vi "CAN.Initialize.vi"(8 "error in (no error)":errorcluster, 11 "Parameters":T5={"Name"="", "CAN"={"Interface"="", "Baud Rate"=0, "Diagnostic Protocol"=enum."GMLAN", "Transport Protocol"=enum."ISO TP - Normal Mode", "Transmit ID"=0, "Receive ID"=2, "Transmit Extension"=1, "Receive Extension"=255, "Receive UUDT ID"=0, "Enable Stream"=TRUE, "VW TP Channel ID"=1, "Fill Frame"=FALSE, "Fill Byte"=0, "Termination"=FALSE, "LIN Cluster"="", "NAD"=8, "IO Mode"=0, "Max DLC"=0, "FD Baud Rate"=2, "Timeout"=1}, "986x"={"Enable"=FALSE, "RIO Device"="", "Bitfile"=path ""}, "Reads"=[], "Frames Lookup"=variant(enum16{"GMLAN", "KWP-2000", "UDS"} enum."GMLAN"), "Writes"=[], "DPIDs"=[], "DPID Lookup"=variant(u32 0), "DTC"={"Descriptor"={"DTC Byte Length"=1, "Status Byte Length"=1, "Add Data Byte Length"=1, "Byte Order"=enum."Motorola"}, "Value.Code"=[], "Value.String"=[], "Value.J2012String"=[], "Status.Code"=[], "Status.String"=[]}, "Created DTCs"=0, "Polls"=[], "Service Channels Status Lookup"=variant, "Trigger Lookup"=variant, "Security"={"Type"=enum."None", "Source DLL Path"=path "", "Target DLL Path"=path "", "Security Level"=0}} {"Writes"."Signals"."Byte Order" items=["Little Endian", "Big Endian"]; "Writes"."Signals"."Data Type" items=["Signed", "Unsigned", "IEEE Float"]; "CAN"."IO Mode" items=["CAN 2.0", "CAN FD", "CAN FD+BRS"]; "CAN"."Fill Byte" format="%.0x"; "CAN"."VW TP Channel ID" format="%.0x"; "CAN"."Receive UUDT ID" format="%.0x"; "CAN"."Receive Extension" format="%.0x"; "CAN"."Transmit Extension" format="%.0x"; "CAN"."Receive ID" format="%.0x"; "CAN"."Transmit ID" format="%.0x"; "Reads"."Signals"."Byte Order" items=["Little Endian", "Big Endian"]; "Reads"."Signals"."Data Type" items=["Signed", "Unsigned", "IEEE Float"]}) -> (0 "error out":errorcluster, 1 "ADCS Connection":T22={"Diag CAN Handle"=0, "Transport Protocol"=enum."ISO TP - Normal Mode", "Receive Address Extension"=0, "Transmit Address Extension"=0, "Receive CAN Id"=0, "Transmit CAN Id"=0, "Log Frames ?"=FALSE, "My TP Address"=0, "Other TP Address"=0, "T1"=0, "T2"=0, "T3"=0, "T4"=0, "Tx SN"=0, "Block Size"=0, "Rx SN"=0, "VW TP Initialized?"=FALSE, "Tx block no"=0, "baud rate"=0, "Interface"="", "Channel Diag CAN Handle"=0, "UDP Connection ID"=refnum, "TCP Connection ID"=refnum, "Target IP Addr"=0, "Source Address"=0, "Target Address"=0, "Send Header NACK?"=FALSE, "DLL Handle"=0, "NAD"=0, "Time Stamp read first"=0.0, "Time Stamp read last"=0.0, "Time Stamp write first"=0.0, "Time Stamp write last"=0.0, "Time Stamp write"=0.0, "Time Stamp read"=0.0, " I/O Mode"=0, "FD Baudrate"=0, "TX_DL"=8, "RX_DL"=8, "DoIP Protocol Version"=1, " Selected I/O Mode"=0, "TesterPresent Counter"=0, "TesterPresent Limit"=0, "TesterPresent Tick[ms]"=10, "TesterPresent RequireResponse?"=FALSE, "TesterPresent Stored Ref?"=FALSE, "TesterPresent Message"=[], "TesterPresent Task Handle"=0, "TesterPresent Semaphore"=refnum, "Response Plausibility Check"=1, "Default Version?"=TRUE, "Diagostic Globals"={"Timeout FC (Bs)"=250, "Timeout CF (Cr)"=250, "Timeout Diag Command"=1000, "Receive Block Size (BS)"=0, "Wait Time CF (STmin)"=5, "Max Waits (N_WFTmax)"=10, "Waits to Send (N_WAIT)"=0, "Time between Waits (TW)"=25, "Fill CAN Frames?"=TRUE, "Fill Byte"=255, "Invalid Response as Error?"=FALSE, "Max RspPending Count"=5, "VWTP Command Timeout"=50, "Transport Protocol"=enum."Diagnostics on IP", "Diag CAN Handle"=0, "DLL Handle"=0, "Timeout RspPending"=1000}, "Session-based Properties?"=FALSE} {"Diagostic Globals"."Fill Byte" format="%x"; "TesterPresent Message" format="%.0x"; "Selected I/O Mode" items=["CAN", "CAN FD", "CAN FD+BRS", "ECU Determined"]; "DoIP Protocol Version" items=["2010"=1, "2012"=2]; "RX_DL" items=["8"=8, "12"=12, "16"=16, "20"=20, "24"=24, "32"=32, "48"=48, "64"=64]; "TX_DL" items=["8"=8, "12"=12, "16"=16, "20"=20, "24"=24, "32"=32, "48"=48, "64"=64]; "I/O Mode" items=["CAN", "CAN FD", "CAN FD+BRS", "Not yet determined"]}, 2 "XNET References":T21, 3 "Parameters":T5={"Name"="", "CAN"={"Interface"="", "Baud Rate"=0, "Diagnostic Protocol"=enum."GMLAN", "Transport Protocol"=enum."ISO TP - Normal Mode", "Transmit ID"=0, "Receive ID"=2, "Transmit Extension"=1, "Receive Extension"=255, "Receive UUDT ID"=0, "Enable Stream"=TRUE, "VW TP Channel ID"=1, "Fill Frame"=FALSE, "Fill Byte"=0, "Termination"=FALSE, "LIN Cluster"="", "NAD"=8, "IO Mode"=0, "Max DLC"=0, "FD Baud Rate"=2, "Timeout"=1}, "986x"={"Enable"=FALSE, "RIO Device"="", "Bitfile"=path ""}, "Reads"=[], "Frames Lookup"=variant(enum16{"GMLAN", "KWP-2000", "UDS"} enum."GMLAN"), "Writes"=[], "DPIDs"=[], "DPID Lookup"=variant(u32 0), "DTC"={"Descriptor"={"DTC Byte Length"=1, "Status Byte Length"=1, "Add Data Byte Length"=1, "Byte Order"=enum."Motorola"}, "Value.Code"=[], "Value.String"=[], "Value.J2012String"=[], "Status.Code"=[], "Status.String"=[]}, "Created DTCs"=0, "Polls"=[], "Service Channels Status Lookup"=variant, "Trigger Lookup"=variant, "Security"={"Type"=enum."None", "Source DLL Path"=path "", "Target DLL Path"=path "", "Security Level"=0}} {"Writes"."Signals"."Byte Order" items=["Little Endian", "Big Endian"]; "Writes"."Signals"."Data Type" items=["Signed", "Unsigned", "IEEE Float"]; "CAN"."IO Mode" items=["CAN 2.0", "CAN FD", "CAN FD+BRS"]; "CAN"."Fill Byte" format="%.0x"; "CAN"."VW TP Channel ID" format="%.0x"; "CAN"."Receive UUDT ID" format="%.0x"; "CAN"."Receive Extension" format="%.0x"; "CAN"."Transmit Extension" format="%.0x"; "CAN"."Receive ID" format="%.0x"; "CAN"."Transmit ID" format="%.0x"; "Reads"."Signals"."Byte Order" items=["Little Endian", "Big Endian"]; "Reads"."Signals"."Data Type" items=["Signed", "Unsigned", "IEEE Float"]}, 5 "Stream Refs":T1 {"Termination" items=["Off", "On"]})   [LabVIEW 2019, in "Diagnostics Addon Engine.lvlib"]
uses:
  Diagnostics Addon Engine.lvlib
  Addon Shared/Types/SysDef.Compile.ctl
  Addon Shared/Types/CAN.ctl
  Addon Shared/Types/CAN.Interface.ctl
  Addon Shared/Types/Protocol.ctl
  Addon Shared/Types/Transport.ctl
  Addon Shared/Types/986x.ctl
  Addon Shared/Types/Frame.Compile.ctl
  Addon Shared/Types/Type.ctl
  Addon Shared/Types/Signal.ctl
  Addon Shared/Types/DPID.ctl
  Addon Shared/Types/DPID.Rate.ctl
  Addon Shared/Types/DTC.Settings.ctl
  Addon Shared/Types/DTC.Descriptor.ctl
  Addon Shared/Types/Poll.Compiled.ctl
  Addon Shared/Types/Security.ctl
  Addon Shared/Types/Security.Type.ctl
  <vilib>/Automotive Diagnostic Command Set/Diagnostic Transport.llb/Diag Reference.ctl
  <vilib>/Automotive Diagnostic Command Set/Diagnostic Transport.llb/Transport Protocol Selector.ctl
  <vilib>/Automotive Diagnostic Command Set/Diagnostic Transport.llb/DoIP Protocol Version.ctl
  <vilib>/Automotive Diagnostic Command Set/Diagnostic Transport.llb/Diag Globals.ctl
  Types/XNET.Refs.ctl
  SubModules/CAN-Streaming-Support/Addon/Addon Engine/Types/Engine Stream Refs.ctl
  SubModules/CAN-Streaming-Support/Addon/Addon Shared/Types/Direction Filter.ctl
  SubModules/CAN-Streaming-Support/Addon/Addon Shared/Types/Type Filter.ctl
  SubModules/CAN-Streaming-Support/Addon/Addon Shared/Types/Filter Parameters.ctl
  <vilib>/xnet/xnet.llb/XNET Create Session (Frame Input Queued).vi
  SubModules/CAN-Streaming-Support/Addon/Addon Engine/CAN Stream Support Engine.lvlib
  Addon Shared/Diagnostics Addon Shared.lvlib
  <vilib>/addons/Automotive Diagnostic Command Set/NI_Automotive Diagnostic Command Set.lvlib
  SubModules/CAN-Streaming-Support/Addon/Addon Shared/CAN Stream Support Shared.lvlib
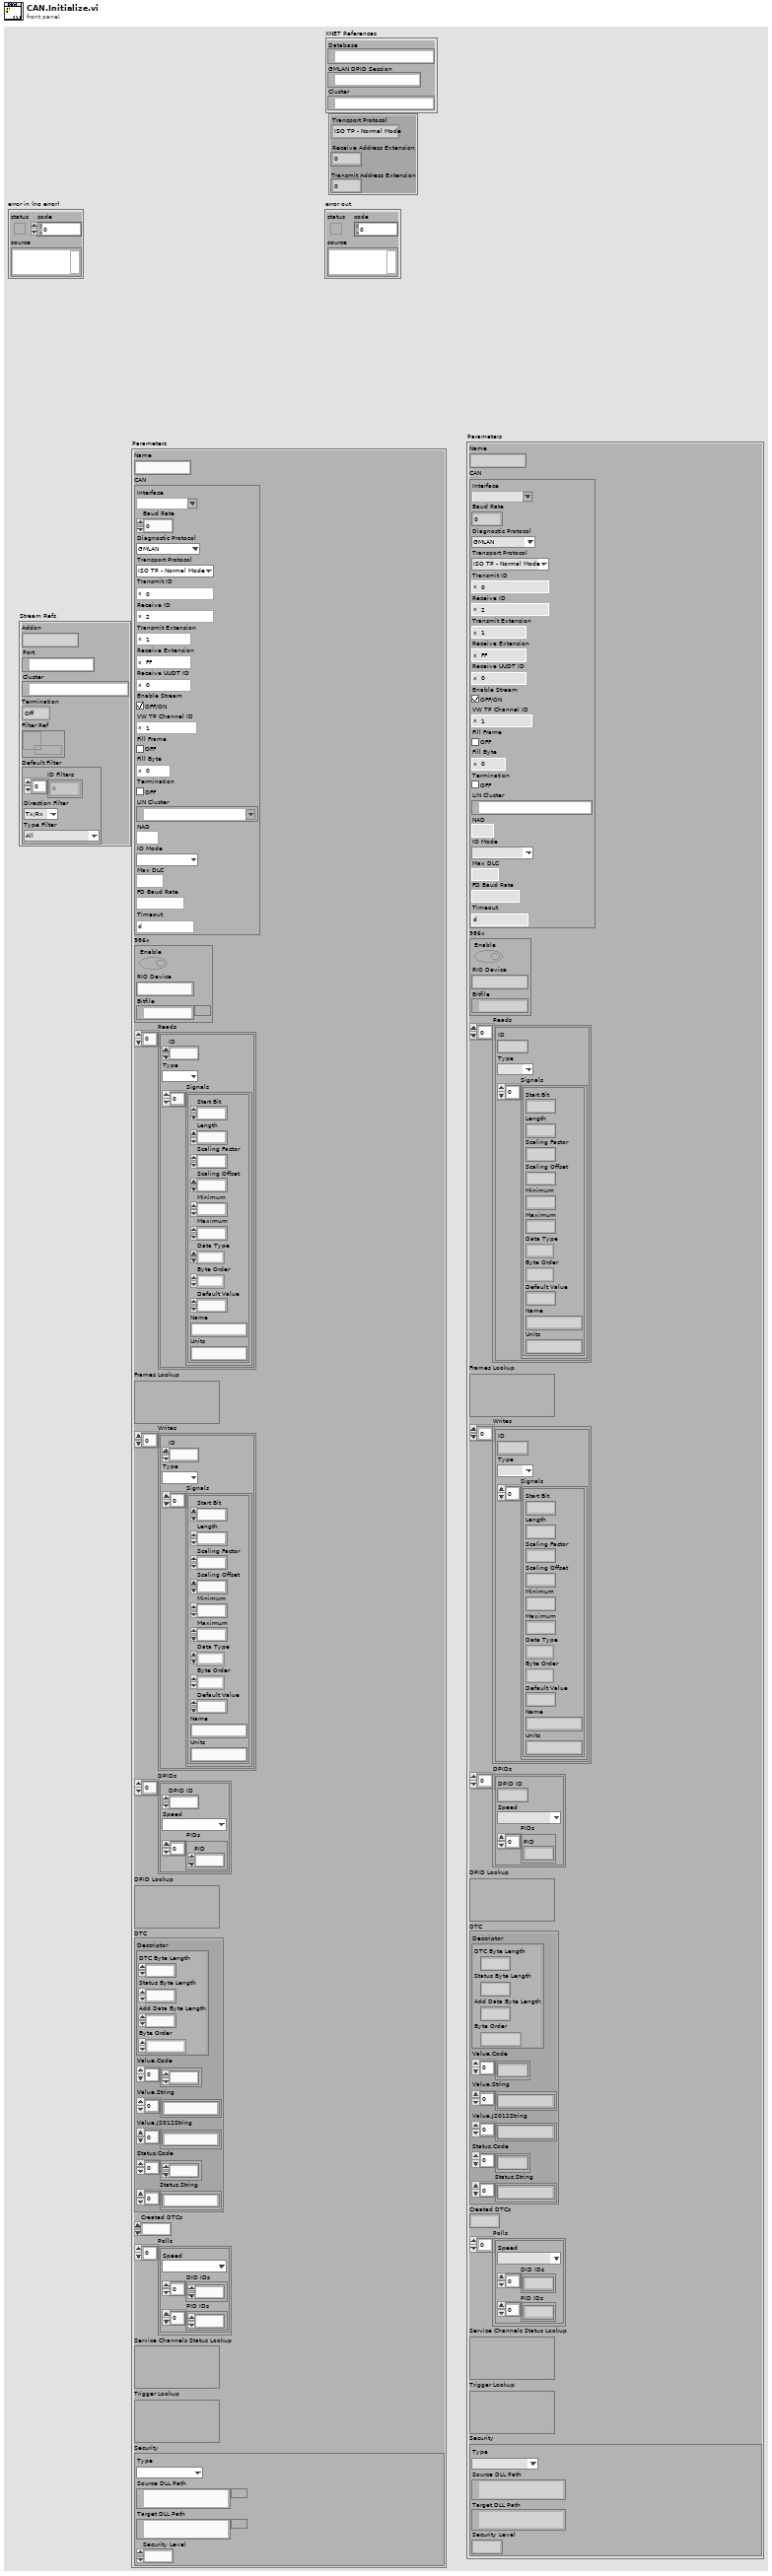
[diagram p1: front panel]
types:
  T1 = typedef "CAN Stream Support Engine.lvlib/Engine Stream Refs.ctl" = cluster{"Addon":string, "Port":refnum<k21>, "Cluster":refnum<k21>, "Termination":u32, "Filter Ref":refnum<data-value>, "Default Filter":T2}
  T2 = typedef "CAN Stream Support Shared.lvlib/Filter Parameters.ctl" = cluster{"ID Filters":u32[], "Direction Filter":T3, "Type Filter":T4}
  T3 = typedef "CAN Stream Support Shared.lvlib/Direction Filter.ctl" = enum16{"Tx/Rx", "Rx", "Tx"}
  T4 = typedef "CAN Stream Support Shared.lvlib/Type Filter.ctl" = enum16{"All", "CAN Data", "CAN Remote", "CAN Bus Error", "CAN 2.0 Data", "CAN FD Data", "CAN FD+BRS Data", "J1939 Data", "Delay", "Log Trigger", "Start Trigger"}
  T5 = typedef "Diagnostics Addon Shared.lvlib/SysDef.Compile.ctl" = cluster{"Name":string, "CAN":T6, "986x":T10, "Reads":T11[], "Frames Lookup":variant, "Writes":T11[], "DPIDs":T14[], "DPID Lookup":variant, "DTC":T16, "Created DTCs":u32, "Polls":T18[], "Service Channels Status Lookup":variant, "Trigger Lookup":variant, "Security":T19}
  T6 = typedef "Diagnostics Addon Shared.lvlib/CAN.ctl" = cluster{"Interface":T7, "Baud Rate":u64, "Diagnostic Protocol":T8, "Transport Protocol":T9, "Transmit ID":u32, "Receive ID":u32, "Transmit Extension":u8, "Receive Extension":u8, "Receive UUDT ID":u32, "Enable Stream":bool, "VW TP Channel ID":u32, "Fill Frame":bool, "Fill Byte":u8, "Termination":bool, "LIN Cluster":refnum<k21>, "NAD":u8, "IO Mode":u32, "Max DLC":u16, "FD Baud Rate":u64, "Timeout":u32}
  T7 = typedef "Diagnostics Addon Shared.lvlib/CAN.Interface.ctl" = string
  T8 = typedef "Diagnostics Addon Shared.lvlib/Protocol.ctl" = enum16{"GMLAN", "KWP-2000", "UDS", "User-Defined"}
  T9 = typedef "Diagnostics Addon Shared.lvlib/Transport.ctl" = enum16{"ISO TP - Normal Mode", "ISO TP - Mixed Mode", "VW TP 2.0", "Diagnostics on IP", "ISO TP LIN"}
  T10 = typedef "Diagnostics Addon Shared.lvlib/986x.ctl" = cluster{"Enable":bool, "RIO Device":string, "Bitfile":path}
  T11 = typedef "Diagnostics Addon Shared.lvlib/Frame.Compile.ctl" = cluster{"ID":u32, "Type":T12, "Signals":T13[]}
  T12 = typedef "Diagnostics Addon Shared.lvlib/Type.ctl" = enum16{"DID", "CDID", "PID", "CPID", "Read Memory", "Write Memory", "IO Control", "Routine Start", "Routine Request", "Routine Stop", "User Defined", "DTC Control", "Clear DTCs", "Read DTCs", "Start DTCs", "DTC Change Count", "Tester Present", "Unlock ECU", "Reset ECU", "Diag Session Control", "Communication Control", "DPID Control", "Poll Control", "Diag CAN Control"}
  T13 = typedef "Diagnostics Addon Shared.lvlib/Signal.ctl" = cluster{"Start Bit":u32, "Length":u32, "Scaling Factor":dbl, "Scaling Offset":dbl, "Minimum":dbl, "Maximum":dbl, "Data Type":u32, "Byte Order":u32, "Default Value":dbl, "Name":string, "Units":string}
  T14 = typedef "Diagnostics Addon Shared.lvlib/DPID.ctl" = cluster{"DPID ID":u8, "Speed":T15, "PIDs":u16[]}
  T15 = typedef "Diagnostics Addon Shared.lvlib/DPID.Rate.ctl" = enum16{"Slow", "Medium", "Fast"}
  T16 = typedef "Diagnostics Addon Shared.lvlib/DTC.Settings.ctl" = cluster{"Descriptor":T17, "Value.Code":dbl[], "Value.String":string[], "Value.J2012String":string[], "Status.Code":dbl[], "Status.String":string[]}
  T17 = typedef "Diagnostics Addon Shared.lvlib/DTC.Descriptor.ctl" = cluster{"DTC Byte Length":i32, "Status Byte Length":i32, "Add Data Byte Length":i32, "Byte Order":enum16{"Motorola", "Intel"}}
  T18 = typedef "Diagnostics Addon Shared.lvlib/Poll.Compiled.ctl" = cluster{"Speed":T15, "DID IDs":u32[], "PID IDs":u32[]}
  T19 = typedef "Diagnostics Addon Shared.lvlib/Security.ctl" = cluster{"Type":T20, "Source DLL Path":path, "Target DLL Path":path, "Security Level":u8}
  T20 = typedef "Diagnostics Addon Shared.lvlib/Security.Type.ctl" = enum16{"None", "DLL", "MasterKey"}
  T21 = typedef "Diagnostics Addon Engine.lvlib/XNET.Refs.ctl" = cluster{"Database":refnum<k21>, "GMLAN DPID Session":refnum<k21>, "Cluster":refnum<k21>}
  T22 = typedef "NI_Automotive Diagnostic Command Set.lvlib/Diag Reference.ctl" = cluster{"Diag CAN Handle":u32, "Transport Protocol":T23, "Receive Address Extension":u8, "Transmit Address Extension":u8, "Receive CAN Id":u32, "Transmit CAN Id":u32, "Log Frames ?":bool, "My TP Address":u8, "Other TP Address":u8, "T1":u16, "T2":u16, "T3":u16, "T4":u16, "Tx SN":u8, "Block Size":u8, "Rx SN":u8, "VW TP Initialized?":bool, "Tx block no":u8, "baud rate":u64, "Interface":string, "Channel Diag CAN Handle":u32, "UDP Connection ID":refnum<k16>, "TCP Connection ID":refnum<k5>, "Target IP Addr":u32, "Source Address":u16, "Target Address":u16, "Send Header NACK?":bool, "DLL Handle":u32, "NAD":u8, "Time Stamp read first":dbl, "Time Stamp read last":dbl, "Time Stamp write first":dbl, "Time Stamp write last":dbl, "Time Stamp write":dbl, "Time Stamp read":dbl, " I/O Mode":u32, "FD Baudrate":u64, "TX_DL":u16, "RX_DL":u16, "DoIP Protocol Version":T24, " Selected I/O Mode":u32, "TesterPresent Counter":u32, "TesterPresent Limit":u32, "TesterPresent Tick[ms]":i32, "TesterPresent RequireResponse?":bool, "TesterPresent Stored Ref?":bool, "TesterPresent Message":u8[], "TesterPresent Task Handle":i32, "TesterPresent Semaphore":T25, "Response Plausibility Check":u32, "Default Version?":bool, "Diagostic Globals":T26, "Session-based Properties?":bool}
  T23 = typedef "NI_Automotive Diagnostic Command Set.lvlib/Transport Protocol Selector.ctl" = enum16{"ISO TP - Normal Mode", "ISO TP - Mixed Mode", "VW TP 2.0", "Diagnostics on IP", "ISO TP LIN"}
  T24 = typedef "NI_Automotive Diagnostic Command Set.lvlib/DoIP Protocol Version.ctl" = u8
  T25 = typedef "Semaphore RefNum" = refnum<k1>
  T26 = typedef "NI_Automotive Diagnostic Command Set.lvlib/Diag Globals.ctl" = cluster{"Timeout FC (Bs)":u32, "Timeout CF (Cr)":u32, "Timeout Diag Command":u32, "Receive Block Size (BS)":u8, "Wait Time CF (STmin)":u8, "Max Waits (N_WFTmax)":u8, "Waits to Send (N_WAIT)":i32, "Time between Waits (TW)":u32, "Fill CAN Frames?":bool, "Fill Byte":u32, "Invalid Response as Error?":bool, "Max RspPending Count":u32, "VWTP Command Timeout":u32, "Transport Protocol":T23, "Diag CAN Handle":u32, "DLL Handle":u32, "Timeout RspPending":u32}
  T27 = enum16{"Output/Write", "Input/Read", "Input/ReadWrite"}
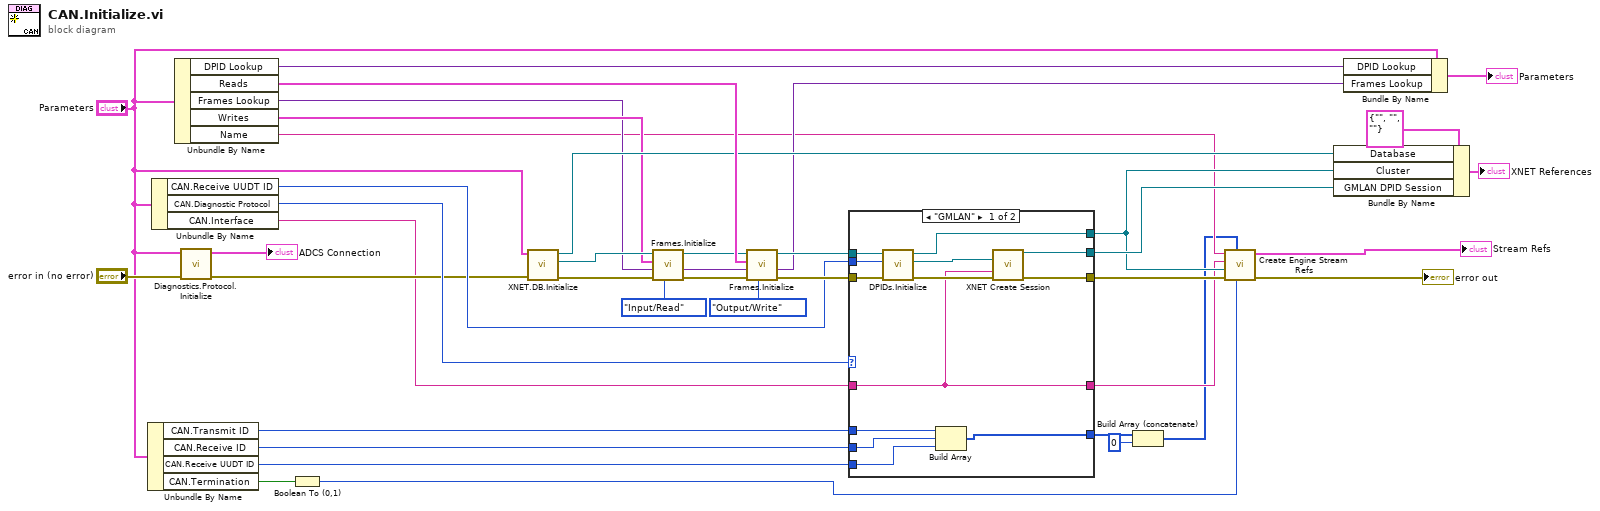
[diagram p0: block diagram]
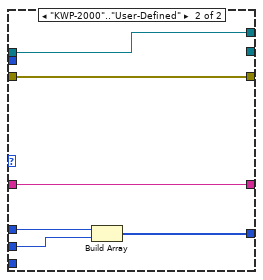
[diagram p2: hidden frame]
diagram:
  n1 = Unbundle By Name("Parameters") -> ("CAN.Transmit ID"=w11:u32, "CAN.Receive ID"=w10:u32, "CAN.Receive UUDT ID"=w9:u32, "CAN.Termination"=w5:bool)
  n2 = Unbundle By Name("Parameters") -> ("CAN.Receive UUDT ID"=w21:u32, "CAN.Diagnostic Protocol"=w22:T8, "CAN.Interface"=w13:T7)
  n3 = Unbundle By Name("Parameters") -> ("DPID Lookup"=w23:variant, "Reads"=w37:T11[], "Frames Lookup"=w25:variant, "Writes"=w27:T11[], "Name"=w6:string)
  n4 = call "Diagnostics.Protocol.Initialize.vi"("error in (no error)"="error in (no error)", "Parameters"="Parameters") -> ("error out"=w20:errorcluster, "diag ref out"=→"ADCS Connection":T22)  [unwired: 8 in]
  n5 = Boolean To (0,1)(Boolean=w5) -> (0, 1=w4:i16)
  n6 = call "XNET.DB.Initialize.vi"("error in (no error)"=w20, "Parameters"="Parameters") -> ("error out"=w28:errorcluster, "Cluster"=w30:refnum<k21>, "XNET Database"=w36:refnum<k21>)  [unwired: 7 in]
  n7 = call "Frames.Initialize.vi"("Direction"=T27."Input/Read", "error in"=w28, "Lookup"=w25, "Frames"=w27, "Cluster In"=w30) -> ("error out"=w26:errorcluster, "Lookup"=w24:variant, "Cluster Out"=w29:refnum<k21>)  [unwired: 4 in]
  n8 = call "Frames.Initialize.vi"("Direction"=T27."Output/Write", "error in"=w26, "Lookup"=w24, "Frames"=w37, "Cluster In"=w29) -> ("error out"=w33:errorcluster, "Lookup"=w31:variant, "Cluster Out"=w32:refnum<k21>)  [unwired: 4 in]
  n9 = case shown="\"GMLAN\"" w22 {
    tunnel: w33 -> [w51 w59]
    tunnel: [w47 w59] -> w16
    tunnel: w13 -> [w45 w57]
    tunnel: w32 -> [w50 w58]
    tunnel: w21 -> [w49 _]
    tunnel: [w48 _] -> w35
    tunnel: [w46 w58] -> w14
    tunnel: [w45 w57] -> w12
    tunnel: w11 -> [w44 w56]
    tunnel: w10 -> [w43 w55]
    tunnel: w9 -> [w42 _]
    tunnel: [w41 w54] -> w2
    frame "GMLAN" {
      n10 = call "DPIDs.Initialize.vi"("error in"=w51, "UUDT Receive ID"=w49, "cluster in"=w50) -> ("error out"=w52:errorcluster, "GMLAN DPID Session"=w53:refnum<k21>, "Cluster Out"=w46:refnum<k21>)  [unwired: 6 in]
      n11 = Build Array(w44, w43, w42) -> (w41:u32[])
      n12 = call-poly <vilib>:"XNET Create Session.vi"("frame"=w53, "interface"=w45, "error in (no error)"=w52) -> ("session out"=w48:refnum<k21>, "error out"=w47:errorcluster)  [unwired: 11 out]
    }
    frame "KWP-2000".."User-Defined" {
      n13 = Build Array(w56, w55) -> (w54:u32[])
    }
  }
  n14 = Build Array (concatenate)(w2, u32 0) -> (w1:u32[])
  n15 = call "Create Engine Stream Refs.vi"("Termination"=w4, "Default IDs"=w1, "error in (no error)"=w16, "Cluster"=w14, "Port"=w12, "Addon"=w6) -> ("error out"=→"error out":errorcluster, "Refs"=→"Stream Refs":T1)  [unwired: 4 in]
  n16 = Bundle By Name(cluster=T21 {"Database"="", "GMLAN DPID Session"="", "Cluster"=""}, "Database"=w36, "Cluster"=w14, "GMLAN DPID Session"=w35) -> (→"XNET References":T21)
  n17 = Bundle By Name(cluster="Parameters", "DPID Lookup"=w23, "Frames Lookup"=w31) -> (→"Parameters":T5)
